vi "Read m1CoverMove.vi"(8 "error in (no error)":errorcluster, 11 "M1Cover in":refnum<class "M1Cover.lvclass">) -> (0 "error out":errorcluster, 2 "coverMoveTypes":T1, 3 "M1Cover out":refnum<class "M1Cover.lvclass">)   [LabVIEW 2014, in "TCSDataDefinitions.lvlib" / "TCSCommand.lvlib" / "M1Cover.lvclass"]
uses:
  M1Cover.lvclass
  Enumerations/M1CoverMoveTypes.ctl
  M1Cover.lvclass/M1Cover.ctl
  TCSCommand.lvlib
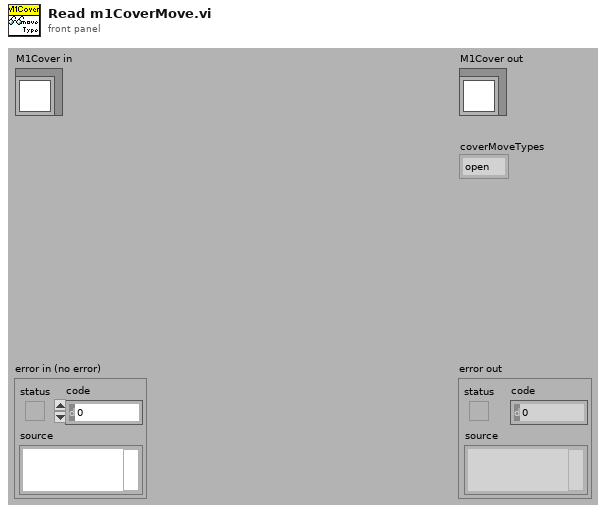
[diagram p1: front panel]
types:
  T1 = typedef "TCSDataDefinitions.lvlib/TCSCommand.lvlib/M1CoverMoveTypes.ctl" = enum16{"open", "close", "stop"}
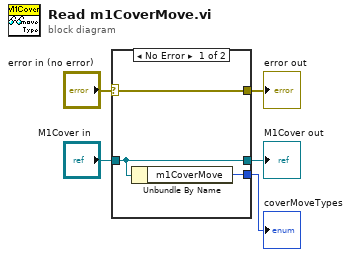
[diagram p0: block diagram]
diagram:
  n1 = case shown="No Error" "error in (no error)" {
    selector: "error in (no error)" -> [w8 w9]
    tunnel: [w8 w9] -> w4
    tunnel: [w7 w10] -> w2
    tunnel: "M1Cover in" -> [w7 w10]
    tunnel: [w6 _] -> w1
    frame No Error {
      n2 = Unbundle By Name(w7) -> ("m1CoverMove"=w6:T1)
    }
    frame Error {
    }
  }
  "error out" <- w4
  "M1Cover out" <- w2
  "coverMoveTypes" <- w1
